vi "Tacking Helper - Final (First) Tack Point.vi"(6 "Intermediate\nWaypoints In":T1[](array[typedef]) {"Point Type" items=["Drive", "Round Port", "Round Starboard", "Stay"]}, 9 "Angle from boat to waypoint":dbl, 10 "End of Array":i32, 11 "Distance to boat":dbl) -> (3 "Intermediate\nWaypoints Out":T1[](array[typedef]) {"Point Type" items=["Drive", "Round Port", "Round Starboard", "Stay"]})   [LabVIEW 2011]
doc: "This vi takes a tack pattern along with the leftover distance to the boat, and extrapolates the angle last used to get the last intermediate waypoint. If done as originally intended, this occurs after all of the jumps, is the only point that doesn't contact the bounding box, and is the closest waypoint to the boat.\n\nTO DO: This vi needs to have at least one jump already completed before it will work - it needs to have a prior angle to go off of."
uses:
  2x3-RIO-OCU Comm/2x3 Typedefs/ocuWaypoint.ctl
  2x3-RIO-OCU Comm/2x3 Typedefs/waypointTypes.ctl
  2 Typedefs/UTM Location.ctl
  <vilib>/Analysis/coordinate.llb/Absolute Angle Difference (scalar).vi
  <vilib>/Analysis/coordinate.llb/Wrap Angle (scalar).vi
  <vilib>/Analysis/coordinate.llb/Set Angle Unit.vi
  <vilib>/Analysis/NI_AAL_Angle.lvlib
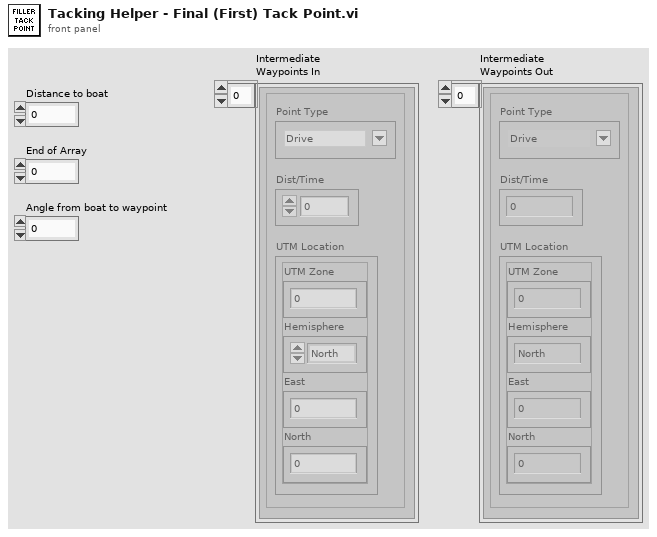
[diagram p1: front panel]
types:
  T1 = typedef "ocuWaypoint.ctl" = cluster{"Point Type":T2, "Dist/Time":dbl, "UTM Location":T3}
  T2 = typedef "waypointTypes.ctl" = u16
  T3 = typedef "UTM Location.ctl" = cluster{"UTM Zone":dbl, "Hemisphere":enum16{"North", "South"}, "East":dbl, "North":dbl}
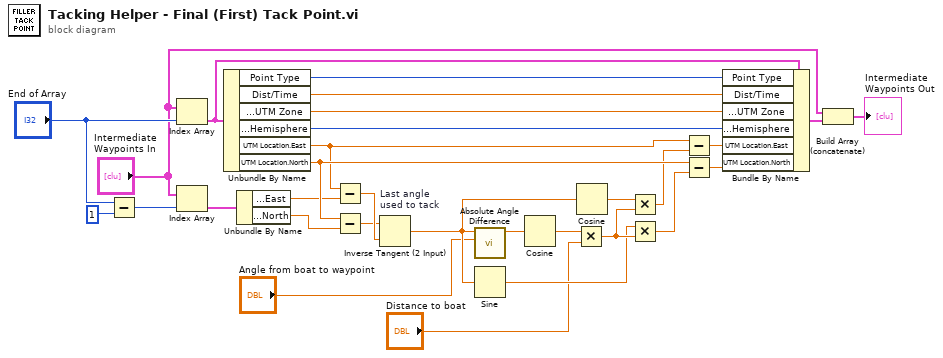
[diagram p0: block diagram]
diagram:
  n1 = Subtract(x="End of Array", y=1) -> (x-y=w10:i32)
  n2 = Index Array(array="Intermediate\nWaypoints In", index="End of Array") -> (element=w2:T1)
  n3 = Index Array(array="Intermediate\nWaypoints In", index=w10) -> (element=w11:T1)
  n4 = Unbundle By Name(w2) -> ("Point Type"=w4:T2, "Dist/Time"=w5:dbl, "UTM Location.UTM Zone"=w6:dbl, "UTM Location.Hemisphere"=w7:enum16{"North", "South"}, "UTM Location.East"=w28:dbl, "UTM Location.North"=w29:dbl)
  n5 = Unbundle By Name(w11) -> ("UTM Location.East"=w27:dbl, "UTM Location.North"=w30:dbl)
  n6 = Subtract(x=w28, y=w27) -> (x-y=w13:dbl)
  n7 = Subtract(x=w29, y=w30) -> (x-y=w12:dbl)
  n8 = Inverse Tangent (2 Input) "Last angle\nused to tack"(1:w13, 2:w12) -> (0:w19:dbl)
  n9 = call-poly <vilib>:"Absolute Angle Difference.vi"("angle 2"="Angle from boat to waypoint", "angle 1"=w19) -> ("absolute angle difference"=w16:dbl)  [unwired: 8 in, 1 out]
  n10 = Sine(x=w19) -> (sin(x)=w21:dbl)
  n11 = Cosine(x=w16) -> (cos(x)=w17:dbl)
  n12 = Multiply(x=w17, y="Distance to boat") -> (x*y=w22:dbl)
  n13 = Cosine(x=w19) -> (cos(x)=w20:dbl)
  n14 = Multiply(x=w20, y=w22) -> (x*y=w23:dbl)
  n15 = Multiply(x=w21, y=w22) -> (x*y=w24:dbl)
  n16 = Subtract(x=w28, y=w23) -> (x-y=w25:dbl)
  n17 = Subtract(x=w29, y=w24) -> (x-y=w26:dbl)
  n18 = Bundle By Name(cluster=w2, "Point Type"=w4, "Dist/Time"=w5, "UTM Location.UTM Zone"=w6, "UTM Location.Hemisphere"=w7, "UTM Location.East"=w25, "UTM Location.North"=w26) -> (w3:T1)
  n19 = Build Array (concatenate)("Intermediate\nWaypoints In", w3) -> (→"Intermediate\nWaypoints Out":T1[])
